vi "Close Data File.vi"(8 "错误输入":errorcluster, 11 "文件引用句柄输入":refnum<file>) -> (0 "错误输出":errorcluster)   [LabVIEW 2012]
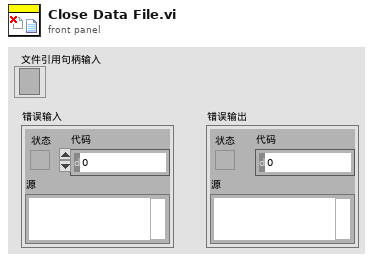
[diagram p1: front panel]
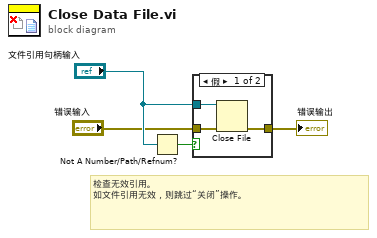
[diagram p0: block diagram]
diagram:
  # "检查无效引用。\n如文件引用无效，则跳过“关闭”操作。"
  n1 = Not A Number/Path/Refnum? ("非法数字/路径/引用句柄？")(number/path/refnum="文件引用句柄输入") -> (NaN/Path/Refnum?=w4:bool)
  n2 = case shown="假" w4 {
    tunnel: "错误输入" -> [w7 w8]
    tunnel: "文件引用句柄输入" -> [w6 _]
    tunnel: [w5 w8] -> w2
    frame False {
      n3 = Close File ("关闭文件")(refnum=w6, error in=w7) -> (error out=w5:errorcluster)  [unwired: 1 out]
    }
    frame True {
    }
  }
  "错误输出" <- w2
